vi "DeviceOpen.vi"(8 "error in (no error)":errorcluster, 10 "Delay between send and receive [ms]":i32=100, 11 "SCD in":refnum<class "SCD.lvclass">) -> (0 "error out":errorcluster, 1 "ID":i32, 2 "device is open?":bool, 3 "SCD out":refnum<class "SCD.lvclass">)   [LabVIEW 2023, in "SCD.lvclass"]
uses:
  SCD.lvclass
  GenericDevice/GenericDevice.lvclass
  SCD.lvclass/SCD.ctl
panel:
  # "Connector Pane"
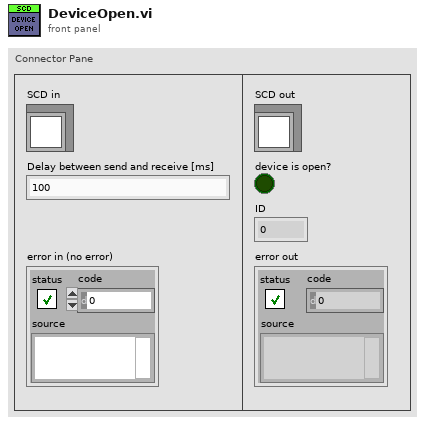
[diagram p1: front panel]
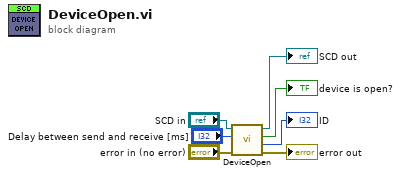
[diagram p0: block diagram]
diagram:
  n1 = call-parent "DeviceOpen.vi"("error in (no error)"="error in (no error)", "Delay between send and receive [ms]"="Delay between send and receive [ms]", "GenericDevice in"="SCD in") -> ("error out"=→"error out":errorcluster, "ID"=→"ID":i32, "device is open?"=→"device is open?":bool, "GenericDevice out"=→"SCD out":refnum<class "SCD.lvclass">)  [unwired: 5 in]
